vi "호출대상.vi"(6 "dB On (F)":bool=TRUE caption="dB On (거짓)", 8 "window":T2=1 caption="윈도우" items=["사각형"=0, "해닝"=1, "해밍"=2, "블랙맨-해리스"=3, "정밀한 블랙맨"=4, "블랙맨"=5, "플랫 탑(Flat Top)"=6, "4항 블랙맨-해리스 "=7, "7항 블랙맨-해리스"=8, "낮은 사이드로브"=9, "블랙맨 누탈"=11, "삼각파"=30, "바틀렛-해닝"=31, "보먼"=32, "파젠"=33, "웰치"=34, "카이저"=60, "돌프-체비셰프"=61, "가우스"=62], 9 "export mode":T1 caption="반출 모드" items=["파워 스펙트럼", "파워 스펙트럼 밀도"], 10 "frequency":dbl=10.0 caption="주파수" format="%0.2p", 11 "signal type":T3(ring) caption="신호 타입") -> (2 "웨이브폼 그래프":cluster{"f0":dbl, "df":dbl, "magnitude":dbl[]}(graph))   [LabVIEW 2014]
uses:
  <vilib>/Analysis/4window.llb/windowTd.ctl
  <vilib>/measure/maspectr.llb/Power Spectrum and PSD Export Mode.ctl
  <vilib>/measure/maspectr.llb/FFT Power Spectrum and PSD for 1 Chan.vi
  <vilib>/measure/NI_MABase.lvlib
  <vilib>/measure/NI_MAPro.lvlib
  <vilib>/Analysis/NI_AALPro.lvlib
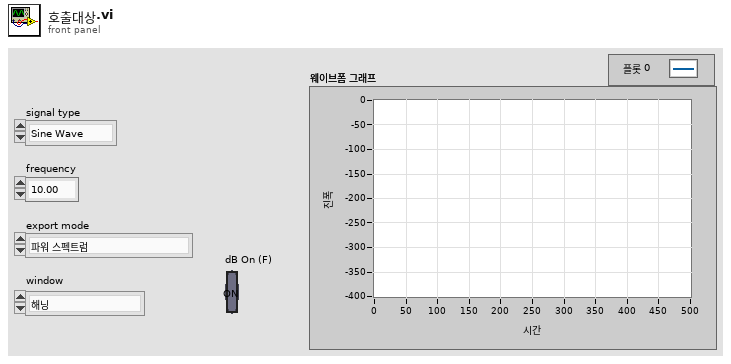
[diagram p1: front panel]
types:
  T1 = typedef "NI_MAPro.lvlib/Power Spectrum and PSD Export Mode.ctl" = u16
  T2 = typedef "NI_AALPro.lvlib/windowTd.ctl" = u32
  T3 = enum16{"Sine Wave", "Triangle Wave", "Square Wave", "Sawtooth Wave"}
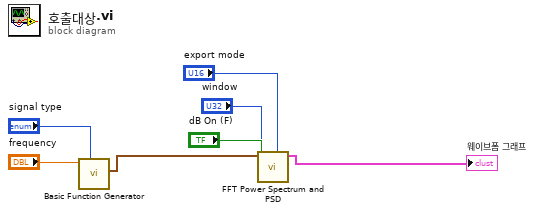
[diagram p0: block diagram]
diagram:
  n1 = call <vilib>:"Basic Function Generator.vi"("signal type"="signal type", "frequency"="frequency") -> ("signal out"=w1:waveform(dbl))  [unwired: 7 in, 2 out]
  n2 = call-poly <vilib>:"FFT Power Spectrum and PSD.vi"("export mode"="export mode", "dB On (F)"="dB On (F)", "window"="window", "time signal"=w1) -> ("Power Spectrum / PSD"=→"웨이브폼 그래프":cluster{"f0":dbl, "df":dbl, "magnitude":dbl[]})  [unwired: 4 in, 3 out]
